vi "Jog btn to Distance.vi"(10 "Distance":dbl[](array[numeric]), 11 "Jog Btn":bool[](array[boolean])) -> (1 "Distance":dbl, 2 "Axis":i32, 3 "Point":string)   [LabVIEW 2019]
panel:
  out "Point Arr":dbl[](array[numeric])
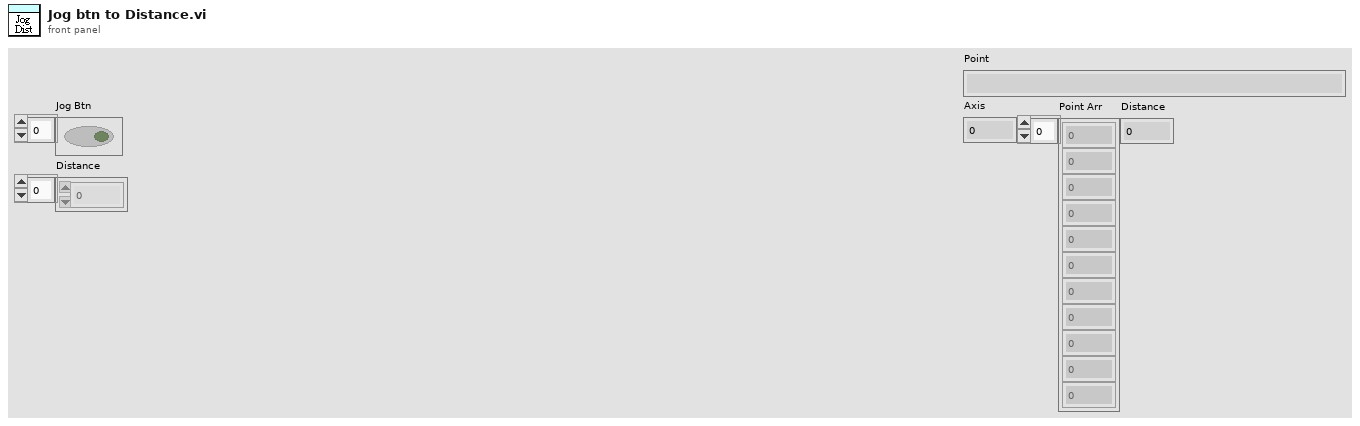
[diagram p1: front panel]
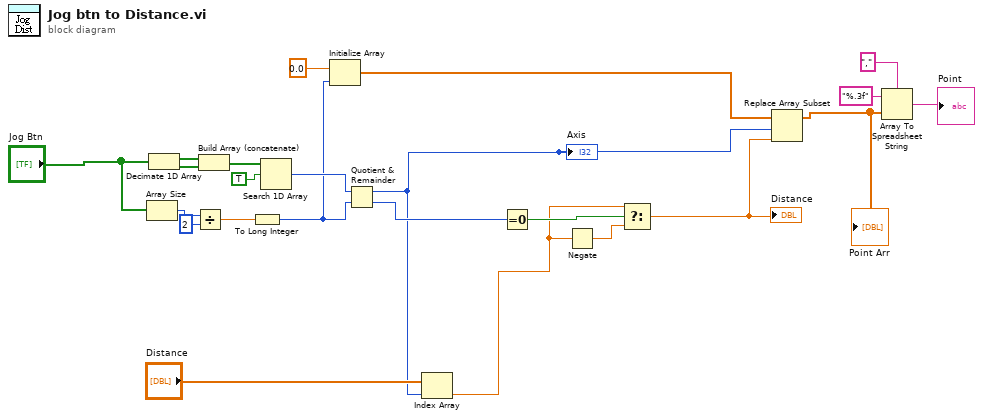
[diagram p0: block diagram]
diagram:
  n1 = Array Size(array="Jog Btn") -> (size(s)=w15:i32)
  n2 = Decimate 1D Array("Jog Btn") -> (w23:bool[], w22:bool[])
  n3 = Divide(x=w15, y=2) -> (x/y=w13:dbl)
  n4 = Build Array (concatenate)(w23, w22) -> (w21:bool[])
  n5 = To Long Integer(number=w13) -> (32bit integer=w12:i32)
  n6 = Search 1D Array(1D array=w21, element=TRUE) -> (index of element=w19:i32)  [unwired: 1 in]
  n7 = Initialize Array(0.0, w12) -> (w10:dbl[])
  n8 = Quotient & Remainder(x=w19, y=w12) -> (x-y*floor(x/y)=w2:i32, floor(x/y)=w18:i32)
  "Axis" <- w2
  n9 = Index Array(array="Distance", index=w2) -> (element=w1:dbl)
  n10 = Equal To 0?(x=w18) -> (x = 0?=w17:bool)
  n11 = Negate(x=w1) -> (-x=w16:dbl)
  n12 = Select(t=w1, s=w17, f=w16) -> (s? t:f=w9:dbl)
  "Distance" <- w9
  n13 = Replace Array Subset(array=w10, new element=w9, index=w2) -> (w8:dbl[])
  "Point Arr" <- w8
  n14 = Array To Spreadsheet String(delimiter (Tab)=",", array=w8, 3:"%.3f" ("format string")) -> (spreadsheet string=→"Point":string)
